vi "SSL_set_cipher_list.vi"(8 "error in (no error)":errorcluster, 10 "Cipher List":string="HIGH:!aNULL:!kRSA:!PSK:!SRP:!MD5:!RC4", 11 "SSL in":refnum<class "SSL.lvclass">) -> (0 "error out":errorcluster, 3 "SSL out":refnum<class "SSL.lvclass">)   [LabVIEW 2013, in "SSL_Lib.lvlib" / "SSL.lvclass"]
uses:
  SSL.lvclass
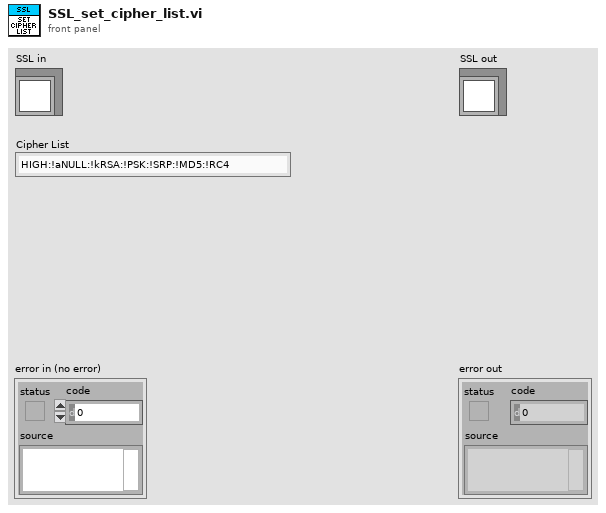
[diagram p1: front panel]
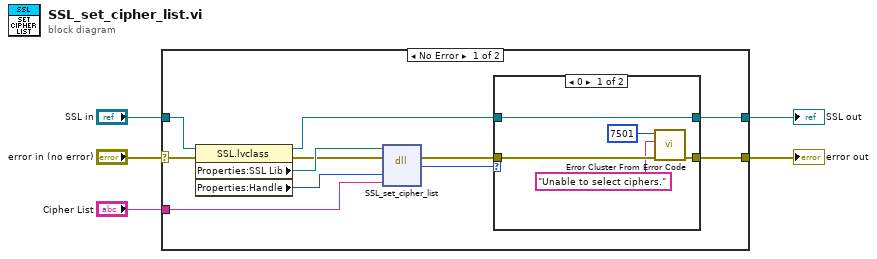
[diagram p0: block diagram]
diagram:
  n1 = case shown="No Error" "error in (no error)" {
    selector: "error in (no error)" -> [w15 w25]
    tunnel: [w11 w25] -> w4
    tunnel: [w9 w24] -> w2
    tunnel: "SSL in" -> [w16 w24]
    tunnel: "Cipher List" -> [w7 _]
    frame No Error {
      n2 = property class="SSL.lvclass"(reference=w16, error in=w15) -> (reference out=w10:refnum<class "SSL.lvclass">, error out=w6:errorcluster, "Properties:SSL Lib"=w13:path, "Properties:Handle"=w14:u64)
      n3 = dll-call lib="C:/Program Files (x86)/National Instruments/Shared/nissl/NIssleay32.dll" fn="SSL_set_cipher_list"(path in=w13, error in=w6, "SSL"=w14, "ciphers"=w7) -> (error out=w12:errorcluster, "return type"=w8:i32)  [unwired: 3 in, 1 out]
      n4 = case shown="0" w8 {
        tunnel: w12 -> [w20 w23]
        tunnel: [w21 w23] -> w11
        tunnel: w10 -> [w19 w22]
        tunnel: [w19 w22] -> w9
        frame 0 {
          n5 = call <vilib>:"Error Cluster From Error Code.vi"("error in (no error)"=w20, "error message (\"\")"="Unable to select ciphers." ("error message (\"\")"), "error code (0)"=7501) -> ("error out"=w21:errorcluster)  [unwired: 6 in]
        }
        frame Default {
        }
      }
    }
    frame Error {
    }
  }
  "error out" <- w4
  "SSL out" <- w2
